vi "sub vi - Calib Lab Panel V1.vi"() -> ()   [LabVIEW 2013]
uses:
  program files/Global display 1.vi
panel:
  in  "Save Button":bool
  out "TIME":string
  out "DATE":string
  out "Temp N":dbl
  out "Temp L":dbl
  out "Power Factor":dbl
  out "VOLTS":dbl
  out "AMPS":dbl
  in  "Select L06 Panel meter":T1(radio)
  in  "CALIBRATION  CERT":T2
  in  "OPEN":bool
  in  "Stop Button":bool
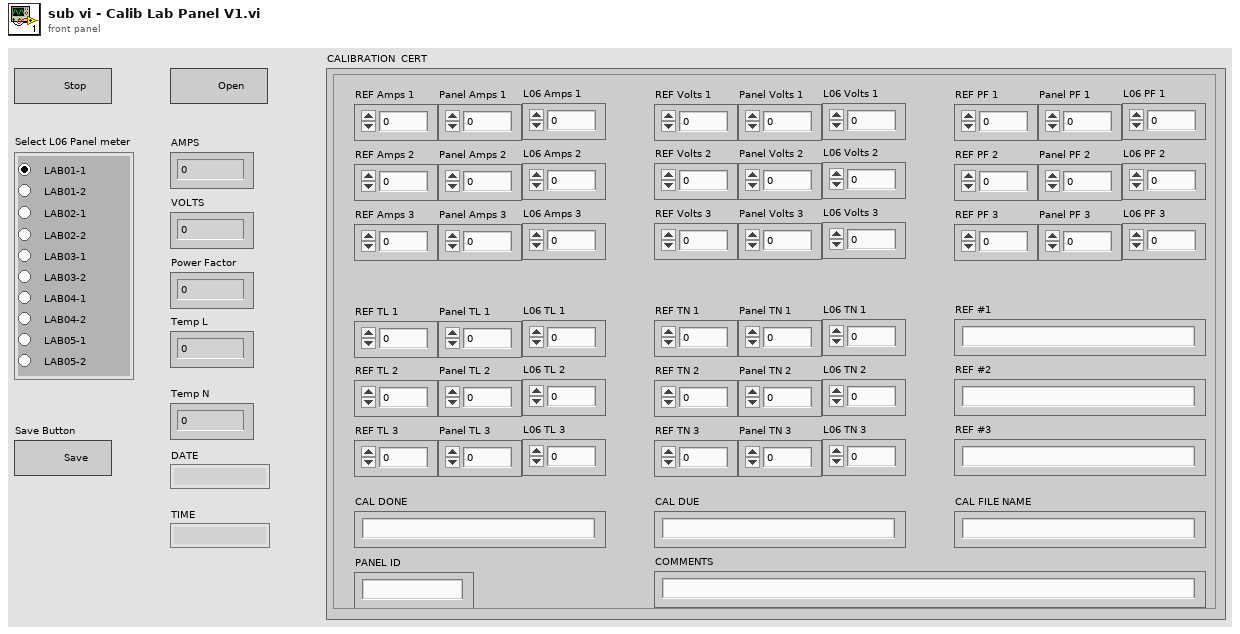
[diagram p1: front panel]
types:
  T1 = enum32{"LAB01-1", "LAB01-2", "LAB02-1", "LAB02-2", "LAB03-1", "LAB03-2", "LAB04-1", "LAB04-2", "LAB05-1", "LAB05-2"}
  T2 = cluster{"REF Amps 1":dbl, "Panel Amps 1":dbl, "L06 Amps 1":dbl, "REF Amps 2":dbl, "Panel Amps 2":dbl, "L06 Amps 2":dbl, "REF Amps 3":dbl, "Panel Amps 3":dbl, "L06 Amps 3":dbl, "REF Volts 1":dbl, "Panel Volts 1":dbl, "L06 Volts 1":dbl, "REF Volts 2":dbl, "Panel Volts 2":dbl, "L06 Volts 2":dbl, "REF Volts 3":dbl, "Panel Volts 3":dbl, "L06 Volts 3":dbl, "REF PF 1":dbl, "Panel PF 1":dbl, "L06 PF 1":dbl, "REF PF 2":dbl, "Panel PF 2":dbl, "L06 PF 2":dbl, "REF PF 3":dbl, "Panel PF 3":dbl, "L06 PF 3":dbl, "REF TL 1":dbl, "Panel TL 1":dbl, "L06 TL 1":dbl, "REF TL 2":dbl, "Panel TL 2":dbl, "L06 TL 2":dbl, "REF TL 3":dbl, "Panel TL 3":dbl, "L06 TL 3":dbl, "REF TN 1":dbl, "Panel TN 1":dbl, "L06 TN 1":dbl, "REF TN 2":dbl, "Panel TN 2":dbl, "L06 TN 2":dbl, "REF TN 3":dbl, "Panel TN 3":dbl, "L06 TN 3":dbl, "REF #1":string, "REF #2":string, "REF #3":string, "CAL DONE":string, "CAL DUE":string, "CAL FILE NAME":string, "COMMENTS":string, "PANEL ID":string}
  T3 = cluster{"AMPS":dbl, "VOLTS":dbl, "PF":dbl, "Tmp Live":dbl, "Tmp Neut":dbl}
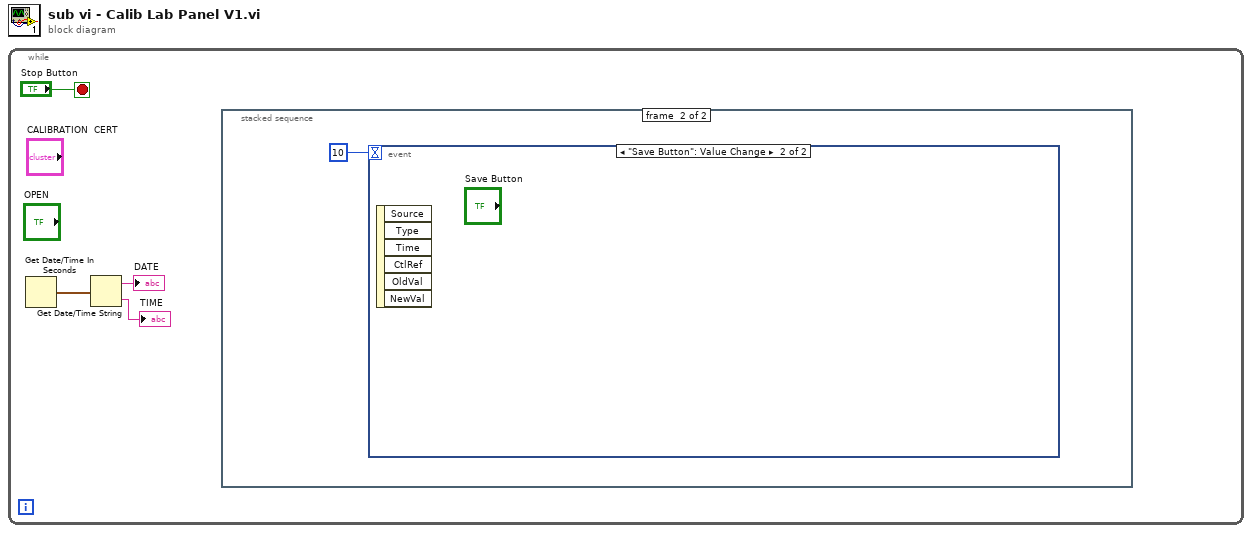
[diagram p0: block diagram]
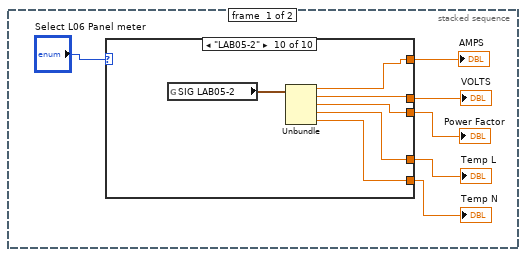
[diagram p2: hidden frame]
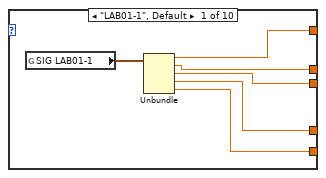
[diagram p3: hidden frame]
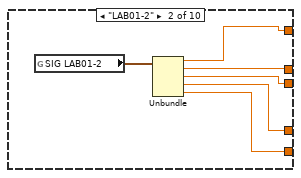
[diagram p4: hidden frame]
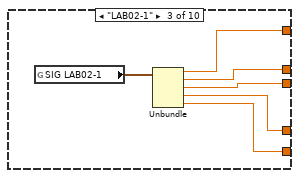
[diagram p5: hidden frame]
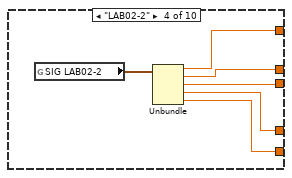
[diagram p6: hidden frame]
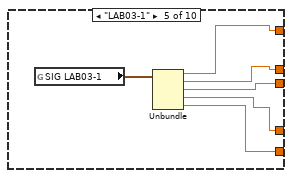
[diagram p7: hidden frame]
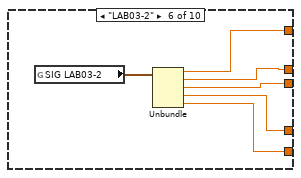
[diagram p8: hidden frame]
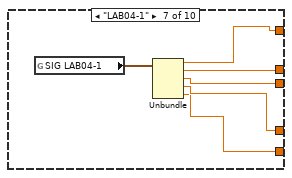
[diagram p9: hidden frame]
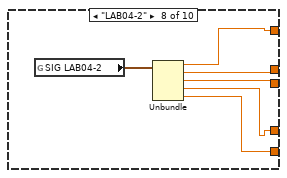
[diagram p10: hidden frame]
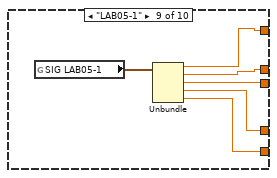
[diagram p11: hidden frame]
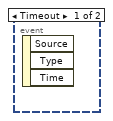
[diagram p12: hidden frame]
diagram:
  n1 = while {
    stop <- "Stop Button" stop-if-true
    n2 = Get Date/Time In Seconds() -> (seconds since 1Jan1904=w3:timestamp)
    n3 = Get Date/Time String(seconds (now)=w3) -> (date string=→"DATE":string, time string=→"TIME":string)  [unwired: 2 in]
    n4 = stacked-sequence {
      frame #0 {
        n5 = case shown="\"LAB05-2\"" "Select L06 Panel meter" {
          tunnel: [w15 w21 w27 w33 w39 w45 w51 w57 w63 w69] -> w9
          tunnel: [w14 w20 w26 w32 w38 w44 w50 w56 w62 w68] -> w8
          tunnel: [w13 w19 w25 w31 w37 w43 w49 w55 w61 w67] -> w7
          tunnel: [w12 w18 w24 w30 w36 w42 w48 w54 w60 w66] -> w6
          tunnel: [w11 w17 w23 w29 w35 w41 w47 w53 w59 w65] -> w5
          frame "LAB01-1", Default {
            n6 = global read "Global display 1.vi" "SIG LAB01-1"() -> (w16:T3)
            n7 = Unbundle(w16) -> ("AMPS"=w15:dbl, "VOLTS"=w14:dbl, "PF"=w13:dbl, "Tmp Live"=w12:dbl, "Tmp Neut"=w11:dbl)
          }
          frame "LAB01-2" {
            n8 = global read "Global display 1.vi" "SIG LAB01-2"() -> (w22:T3)
            n9 = Unbundle(w22) -> ("AMPS"=w21:dbl, "VOLTS"=w20:dbl, "PF"=w19:dbl, "Tmp Live"=w18:dbl, "Tmp Neut"=w17:dbl)
          }
          frame "LAB02-1" {
            n10 = global read "Global display 1.vi" "SIG LAB02-1"() -> (w28:T3)
            n11 = Unbundle(w28) -> ("AMPS"=w27:dbl, "VOLTS"=w26:dbl, "PF"=w25:dbl, "Tmp Live"=w24:dbl, "Tmp Neut"=w23:dbl)
          }
          frame "LAB02-2" {
            n12 = global read "Global display 1.vi" "SIG LAB02-2"() -> (w34:T3)
            n13 = Unbundle(w34) -> ("AMPS"=w33:dbl, "VOLTS"=w32:dbl, "PF"=w31:dbl, "Tmp Live"=w30:dbl, "Tmp Neut"=w29:dbl)
          }
          frame "LAB03-1" {
            n14 = global read "Global display 1.vi" "SIG LAB03-1"() -> (w40:T3)
            n15 = Unbundle(w40) -> ("AMPS"=w39:dbl, "VOLTS"=w38:dbl, "PF"=w37:dbl, "Tmp Live"=w36:dbl, "Tmp Neut"=w35:dbl)
          }
          frame "LAB03-2" {
            n16 = global read "Global display 1.vi" "SIG LAB03-2"() -> (w46:T3)
            n17 = Unbundle(w46) -> ("AMPS"=w45:dbl, "VOLTS"=w44:dbl, "PF"=w43:dbl, "Tmp Live"=w42:dbl, "Tmp Neut"=w41:dbl)
          }
          frame "LAB04-1" {
            n18 = global read "Global display 1.vi" "SIG LAB04-1"() -> (w52:T3)
            n19 = Unbundle(w52) -> ("AMPS"=w51:dbl, "VOLTS"=w50:dbl, "PF"=w49:dbl, "Tmp Live"=w48:dbl, "Tmp Neut"=w47:dbl)
          }
          frame "LAB04-2" {
            n20 = global read "Global display 1.vi" "SIG LAB04-2"() -> (w58:T3)
            n21 = Unbundle(w58) -> ("AMPS"=w57:dbl, "VOLTS"=w56:dbl, "PF"=w55:dbl, "Tmp Live"=w54:dbl, "Tmp Neut"=w53:dbl)
          }
          frame "LAB05-1" {
            n22 = global read "Global display 1.vi" "SIG LAB05-1"() -> (w64:T3)
            n23 = Unbundle(w64) -> ("AMPS"=w63:dbl, "VOLTS"=w62:dbl, "PF"=w61:dbl, "Tmp Live"=w60:dbl, "Tmp Neut"=w59:dbl)
          }
          frame "LAB05-2" {
            n24 = global read "Global display 1.vi" "SIG LAB05-2"() -> (w70:T3)
            n25 = Unbundle(w70) -> ("AMPS"=w69:dbl, "VOLTS"=w68:dbl, "PF"=w67:dbl, "Tmp Live"=w66:dbl, "Tmp Neut"=w65:dbl)
          }
        }
        "AMPS" <- w9
        "VOLTS" <- w8
        "Power Factor" <- w7
        "Temp L" <- w6
        "Temp N" <- w5
      }
      frame #1 {
        n26 = event shown="[1] \"Save Button\": Value Change" {
          selector: _ -> [_ _]
          dyn-events: _ -> [_ _]
          timeout: 10 -> [_ _]
          event Timeout {
            n27 = event-data() -> ()  [unwired: 1 in, 3 out]
          }
          event "Save Button": Value Change {
            n28 = event-data() -> ()  [unwired: 1 in, 6 out]
          }
        }
      }
    }
  }
